vi "my rio lm35.vi"() -> ()   [LabVIEW 2018]
panel:
  out "Filename Out":path
  out "size(s)":i32[](array[numeric])
  out "max value":dbl
  out "Array 3":dbl[][](array[numeric])
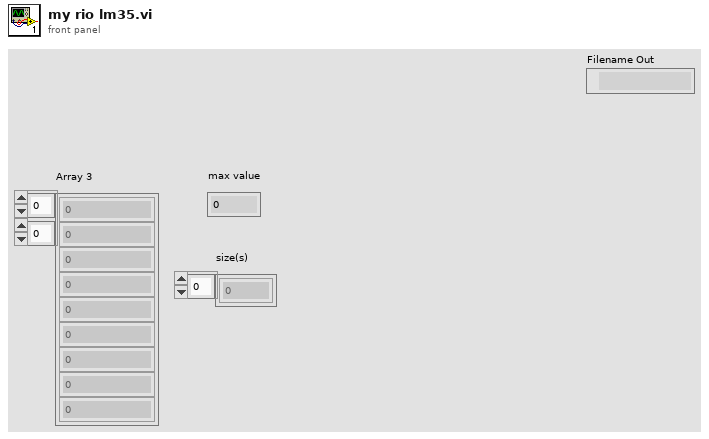
[diagram p1: front panel]
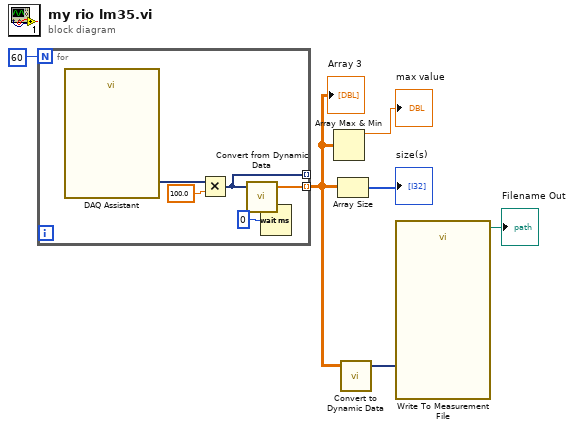
[diagram p0: block diagram]
diagram:
  n1 = for {
    N: 60 -> [_]
    tunnel: [w9] -> _ mode=indexing
    tunnel: [w8] -> w3 mode=indexing
    n2 = call "DAQ Assistant"() -> ("data"=w11:dynamicdata)  [unwired: 17 in, 2 out]
    n3 = Multiply(x=w11, y=100.0) -> (x*y=w9:dynamicdata)
    n4 = call "Convert from Dynamic Data"("Dynamic Data Type"=w9) -> ("Array"=w8:dbl[])  [unwired: 3 in]
    n5 = Wait (ms)(milliseconds to wait=u32 0) -> ()  [unwired: 1 out]
  }
  "Array 3" <- w3
  n6 = Array Max & Min(array=w3) -> (max value=→"max value":dbl)  [unwired: 3 out]
  n7 = Array Size(array=w3) -> (size(s)=→"size(s)":i32[])
  n8 = call "Convert to Dynamic Data"("2D Array"=w3) -> ("Dynamic Data Type"=w2:dynamicdata)  [unwired: 3 in]
  n9 = call "Write To Measurement File"("Signals"=w2) -> ("Filename Out"=→"Filename Out":path)  [unwired: 16 in, 2 out]
